vi "PH_SSAC.evt call Remote Control.vi"(0 "i ref in":refnum<vi>, 2 "Instance":string="N/A", 3 "Ctrl Remote?":bool, 5 "error in (no error)":errorcluster) -> (14 "i ref out":refnum<vi>, 19 "error out":errorcluster)   [LabVIEW 2014, in "PH_SSAC.lvlib"]
doc: "This VI sets the instance remotely controlled by a simple call."
uses:
  PH_SSAC.lvlib
  CS_Core/CSSystem/CoreLib/CoreLib.short 2 byte array.vi
  CS_Core/CSSystem/CoreLib/CoreLib.lvlib
  CS_Core/BaseProcess/BaseProcess.lvlib
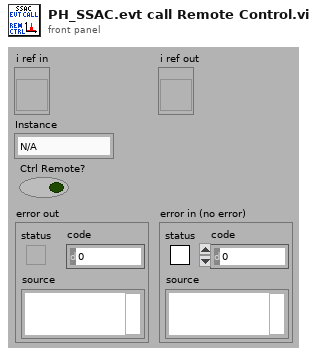
[diagram p1: front panel]
types:
  T1 = typedef "CoreDefs.rawDataType.ctl" = i8[]
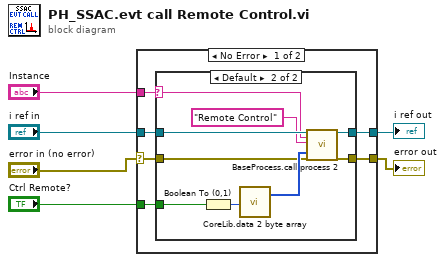
[diagram p0: block diagram]
diagram:
  n1 = case shown="No Error" "error in (no error)" {
    selector: "error in (no error)" -> [w9 w25]
    tunnel: [w12 w24] -> w6
    tunnel: [w11 w25] -> w5
    tunnel: "i ref in" -> [w10 w24]
    tunnel: "Instance" -> [w8 _]
    tunnel: "Ctrl Remote?" -> [w7 _]
    frame No Error {
      n2 = case shown="Default" w8 {
        selector: w8 -> [_ w16]
        tunnel: [w14 w23] -> w12
        tunnel: [w13 w22] -> w11
        tunnel: w10 -> [w14 w21]
        tunnel: w9 -> [w13 w17]
        tunnel: w7 -> [_ w15]
        frame "N/A" {
        }
        frame Default {
          n3 = Boolean To (0,1)(Boolean=w15) -> (0, 1=w19:i16)
          n4 = call-poly "CoreLib.data 2 byte array.vi"("i16"=w19) -> ("byteArray out"=w18:T1)  [unwired: 18 in]
          n5 = call "BaseProcess.call process 2.vi"("i ref in"=w21, "Object"=w16, "Selector"="Remote Control", "Data"=w18, "error in (no error)"=w17) -> ("i ref out"=w23:refnum<vi>, "error out"=w22:errorcluster)  [unwired: 13 in]
        }
      }
    }
    frame Error {
    }
  }
  "error out" <- w5
  "i ref out" <- w6
